vi "Additive Colour Mixer.vi"(8 "error in (no error)":errorcluster, 11 "Colours":u32[](array[colorbox])) -> (0 "error out":errorcluster, 3 "Mixed colour":u32(colorbox)=16777216)   [LabVIEW 2018, in "Colour Lab.lvlib"]
uses:
  Colour Lab.lvlib
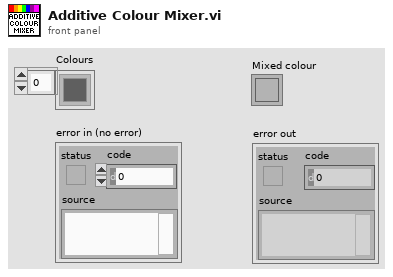
[diagram p1: front panel]
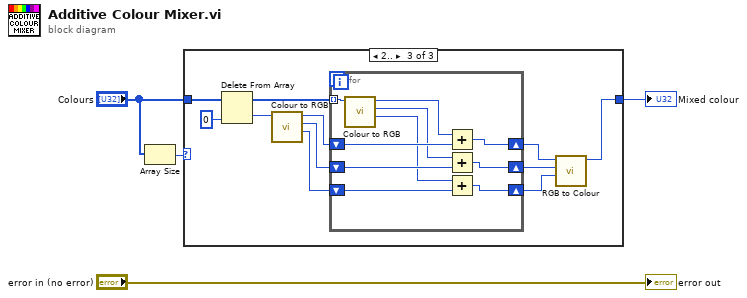
[diagram p0: block diagram]
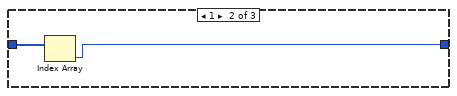
[diagram p3: hidden frame]
diagram:
  n1 = Array Size(array="Colours") -> (size(s)=w2:i32)
  n2 = case shown="2.." w2 {
    tunnel: "Colours" -> [_ w6 w16]
    tunnel: [_ w5 w10] -> w1
    frame ..0 {
    }
    frame 1 {
      n3 = Index Array(array=w6) -> (element=w5:u32)  [unwired: 1 in]
    }
    frame 2.. {
      n4 = Delete From Array(array=w16, index=0) -> (deleted portion=w15:u32, array with subset deleted=w14:u32[])  [unwired: 1 in]
      n5 = call "Colour to RGB.vi"("Colour"=w15) -> ("Blue"=w13:u8, "Green"=w12:u8, "Red"=w11:u8)  [unwired: 6 in, 2 out]
      n6 = for {
        shift-right: [w22] -> w9
        shift-left: w11 -> [w24]
        tunnel: w14 -> [w27] mode=indexing
        shift-right: [w23] -> w8
        shift-left: w12 -> [w25]
        shift-right: [w21] -> w7
        shift-left: w13 -> [w26]
        n7 = call "Colour to RGB.vi"("Colour"=w27) -> ("Blue"=w18:u8, "Green"=w19:u8, "Red"=w20:u8)  [unwired: 6 in, 2 out]
        n8 = Add(x=w20, y=w24) -> (x+y=w22:u8)
        n9 = Add(x=w19, y=w25) -> (x+y=w23:u8)
        n10 = Add(x=w18, y=w26) -> (x+y=w21:u8)
      }
      n11 = call "RGB to Colour.vi"("Blue"=w7, "Green"=w8, "Red"=w9) -> ("Color"=w10:u32)  [unwired: 7 in, 1 out]
    }
  }
  "Mixed colour" <- w1
  "error out" <- "error in (no error)"
